vi "From bytes.vi"(8 "error in (no error)":errorcluster, 11 "Bytes in":u8[](array[numeric]) format="%x") -> (0 "error out":errorcluster, 1 "Boolean":bool, 2 "MsgPackBool out":refnum<class "MsgPackBool.lvclass">, 3 "remaining bytes":u8[](array[numeric]))   [LabVIEW 2020, in "MessagePack.lvlib" / "MsgPackBool.lvclass"]
uses:
  MsgPackBool.lvclass
  MessagePack.lvlib
  <vilib>/Utility/error.llb/Error Cluster From Error Code.vi
  <vilib>/ErrorRing/Error Ring.xnode
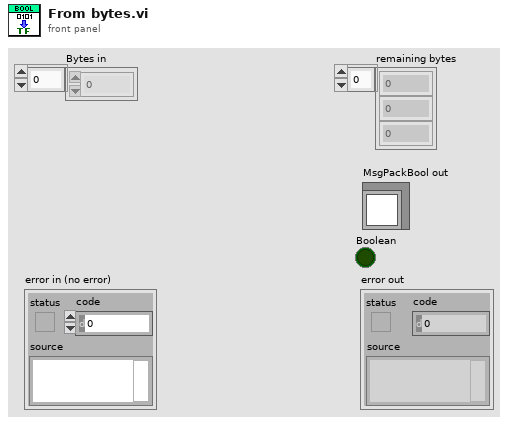
[diagram p1: front panel]
types:
  T1 = typedef "MessagePack.lvlib/MsgPack Object Types.ctl" = enum16{"UNSUPPORTED", "POSINT", "NEGINT", "FIXMAP", "FIXARRAY", "FIXSTR", "NIL", "FALSE", "TRUE", "BIN8", "BIN16", "BIN32", "EXT8", "EXT16", "EXT32", "FLOAT32", "FLOAT64", "UINT8", "UINT16", "UINT32", "UINT64", "INT8", "INT16", "INT32", "INT64", "FIXEXT1", "FIXEXT2", "FIXEXT4", "FIXEXT8", "FIXEXT16", "STR8", "STR16", "STR32", "ARRAY16", "ARRAY32", "MAP16", "MAP32"}
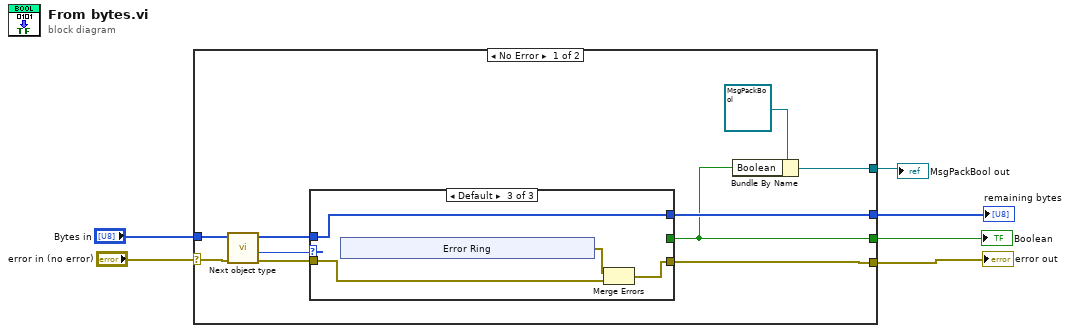
[diagram p0: block diagram]
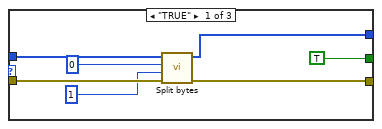
[diagram p2: hidden frame]
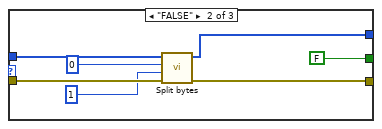
[diagram p3: hidden frame]
diagram:
  n1 = case shown="No Error" "error in (no error)" {
    selector: "error in (no error)" -> [w15 w40]
    tunnel: [w7 w40] -> w5
    tunnel: "Bytes in" -> [w16 w39]
    tunnel: [w11 w39] -> w3
    tunnel: [w9 _] -> w2
    tunnel: [w8 _] -> w1
    frame No Error {
      n2 = call "Next object type.vi"("error in (no error)"=w15, "Bytes in"=w16) -> ("error out"=w13:errorcluster, "MsgPack Type"=w14:T1, "Bytes out"=w12:u8[])  [unwired: 6 in, 1 out]
      n3 = case shown="Default" w14 {
        tunnel: w13 -> [w23 w30 w34]
        tunnel: [w18 w25 w32] -> w7
        tunnel: w12 -> [w20 w27 w31]
        tunnel: [w19 w26 w31] -> w11
        tunnel: [TRUE FALSE _] -> w9
        frame "TRUE" {
          n4 = call "Split bytes.vi"("error in"=w23, "count (1)"=1 ("Count"), "start index (0)"=0 ("Start index"), "bytes in"=w20) -> ("error out"=w18:errorcluster, "remaining bytes"=w19:u8[])  [unwired: 4 in, 2 out]
        }
        frame "FALSE" {
          n5 = call "Split bytes.vi"("error in"=w30, "count (1)"=1 ("Count"), "start index (0)"=0 ("Start index"), "bytes in"=w27) -> ("error out"=w25:errorcluster, "remaining bytes"=w26:u8[])  [unwired: 4 in, 2 out]
        }
        frame Default {
          n6 = xnode "Error Ring"() -> ("error out"=w33:errorcluster)
          n7 = Merge Errors(w33, w34) -> (w32:errorcluster)
        }
      }
      n8 = Bundle By Name(cluster=refnum<class "MsgPackBool.lvclass"> refnum ("MessagePack.lvlib:MsgPackBool.lvclass"), "Boolean"=w9) -> (w8:refnum<class "MsgPackBool.lvclass">)
    }
    frame Error {
    }
  }
  "error out" <- w5
  "MsgPackBool out" <- w1
  "remaining bytes" <- w3
  "Boolean" <- w2
